vi "Live video with note capture.vi"() -> ()   [LabVIEW 2009]
uses:
  <vilib>/vision/Image Controls.llb/IMAQ Image.ctl
  <vilib>/userDefined/High Color/IMAQdx.ctl
  <vilib>/Analysis/3filter.llb/Filter Passband Type.ctl
  <vilib>/Analysis/3filter.llb/Butterworth Filter (DBL).vi
  <vilib>/vision/NI_Vision_Development_Module.lvlib
  <vilib>/Analysis/NI_AALBase.lvlib
  <vilib>/vision/driver/NI_Vision_Acquisition_Software.lvlib
panel:
  in  "frame rate":dbl
  out "Image Dst Out":T1
  out "Blue Line":T2={"Global Rectangle"=[243, 262, 261, 384], "Contours"=[{"ID"=enum."External", "Type"=2, "Coordinates"=[260, 383, 243, 262]}]} {"Contours"."Type" items=["No Selection", "Point", "Line", "Rectangle", "Oval", "Polygon", "Freehand Region", "Annulus", "Unused2", "Unused3", "Broken Line", "Freehand Line", "Rotated Rectangle"]}
  out "Red Line":T2={"Global Rectangle"=[168, 264, 180, 378], "Contours"=[{"ID"=enum."External", "Type"=2, "Coordinates"=[168, 377, 179, 264]}]} {"Contours"."Type" items=["No Selection", "Point", "Line", "Rectangle", "Oval", "Polygon", "Freehand Region", "Annulus", "Unused2", "Unused3", "Broken Line", "Freehand Line", "Rotated Rectangle"]}
  in  "low  2":dbl=0.12500000000000006 format="%0.4f"
  in  "high 2":dbl=60.0 format="%0.2f"
  in  "sampling 2":dbl=1.0 format="%0.2f"
  out "LED BLUE":bool
  out "Waveform BLUE":dbl[](graph)
  out "LED RED":bool
  in  "low":dbl=0.12500000000000006 format="%0.4f"
  out "Waveform RED":dbl[](graph)
  in  "high":dbl=60.0 format="%0.2f"
  in  "sampling":dbl=1.0 format="%0.2f"
  out "Image":T1(plugin-control)
  in  "stop":bool
  # "RED"
  # "BLUE"
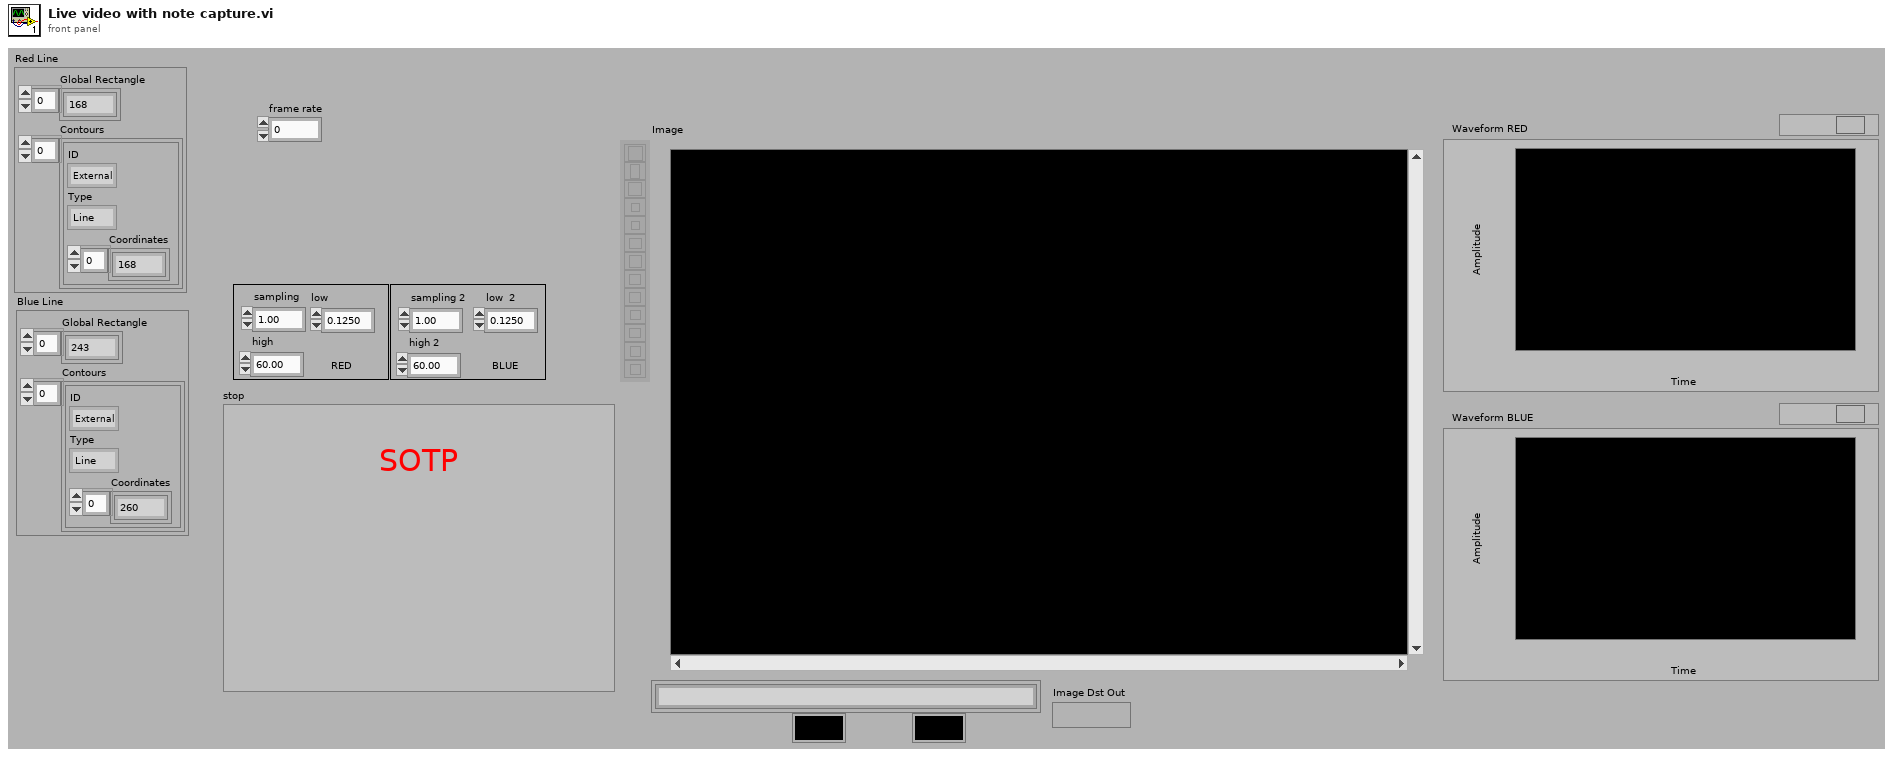
[diagram p1: front panel]
types:
  T1 = typedef "IMAQ Image.ctl" = refnum<image>
  T2 = cluster{"Global Rectangle":i32[], "Contours":cluster{"ID":enum32{"External", "Internal"}, "Type":u32, "Coordinates":i32[]}[]}
  T3 = typedef "IMAQdx.ctl" = refnum<k21>
  T4 = typedef "NI_AALBase.lvlib/Filter Passband Type.ctl" = enum32{"Lowpass", "Highpass", "Bandpass", "Bandstop"}
  T5 = cluster{"Left":i32, "Top":i32, "Right":i32, "Bottom":i32}
  T6 = typedef "Image Type" = u32
  T7 = cluster{"ID":enum32{"External", "Internal"}, "Type":u32, "Coordinates":i32[]}[]
  T8 = cluster{"ID":enum32{"External", "Internal"}, "Type":u32, "Coordinates":i32[]}
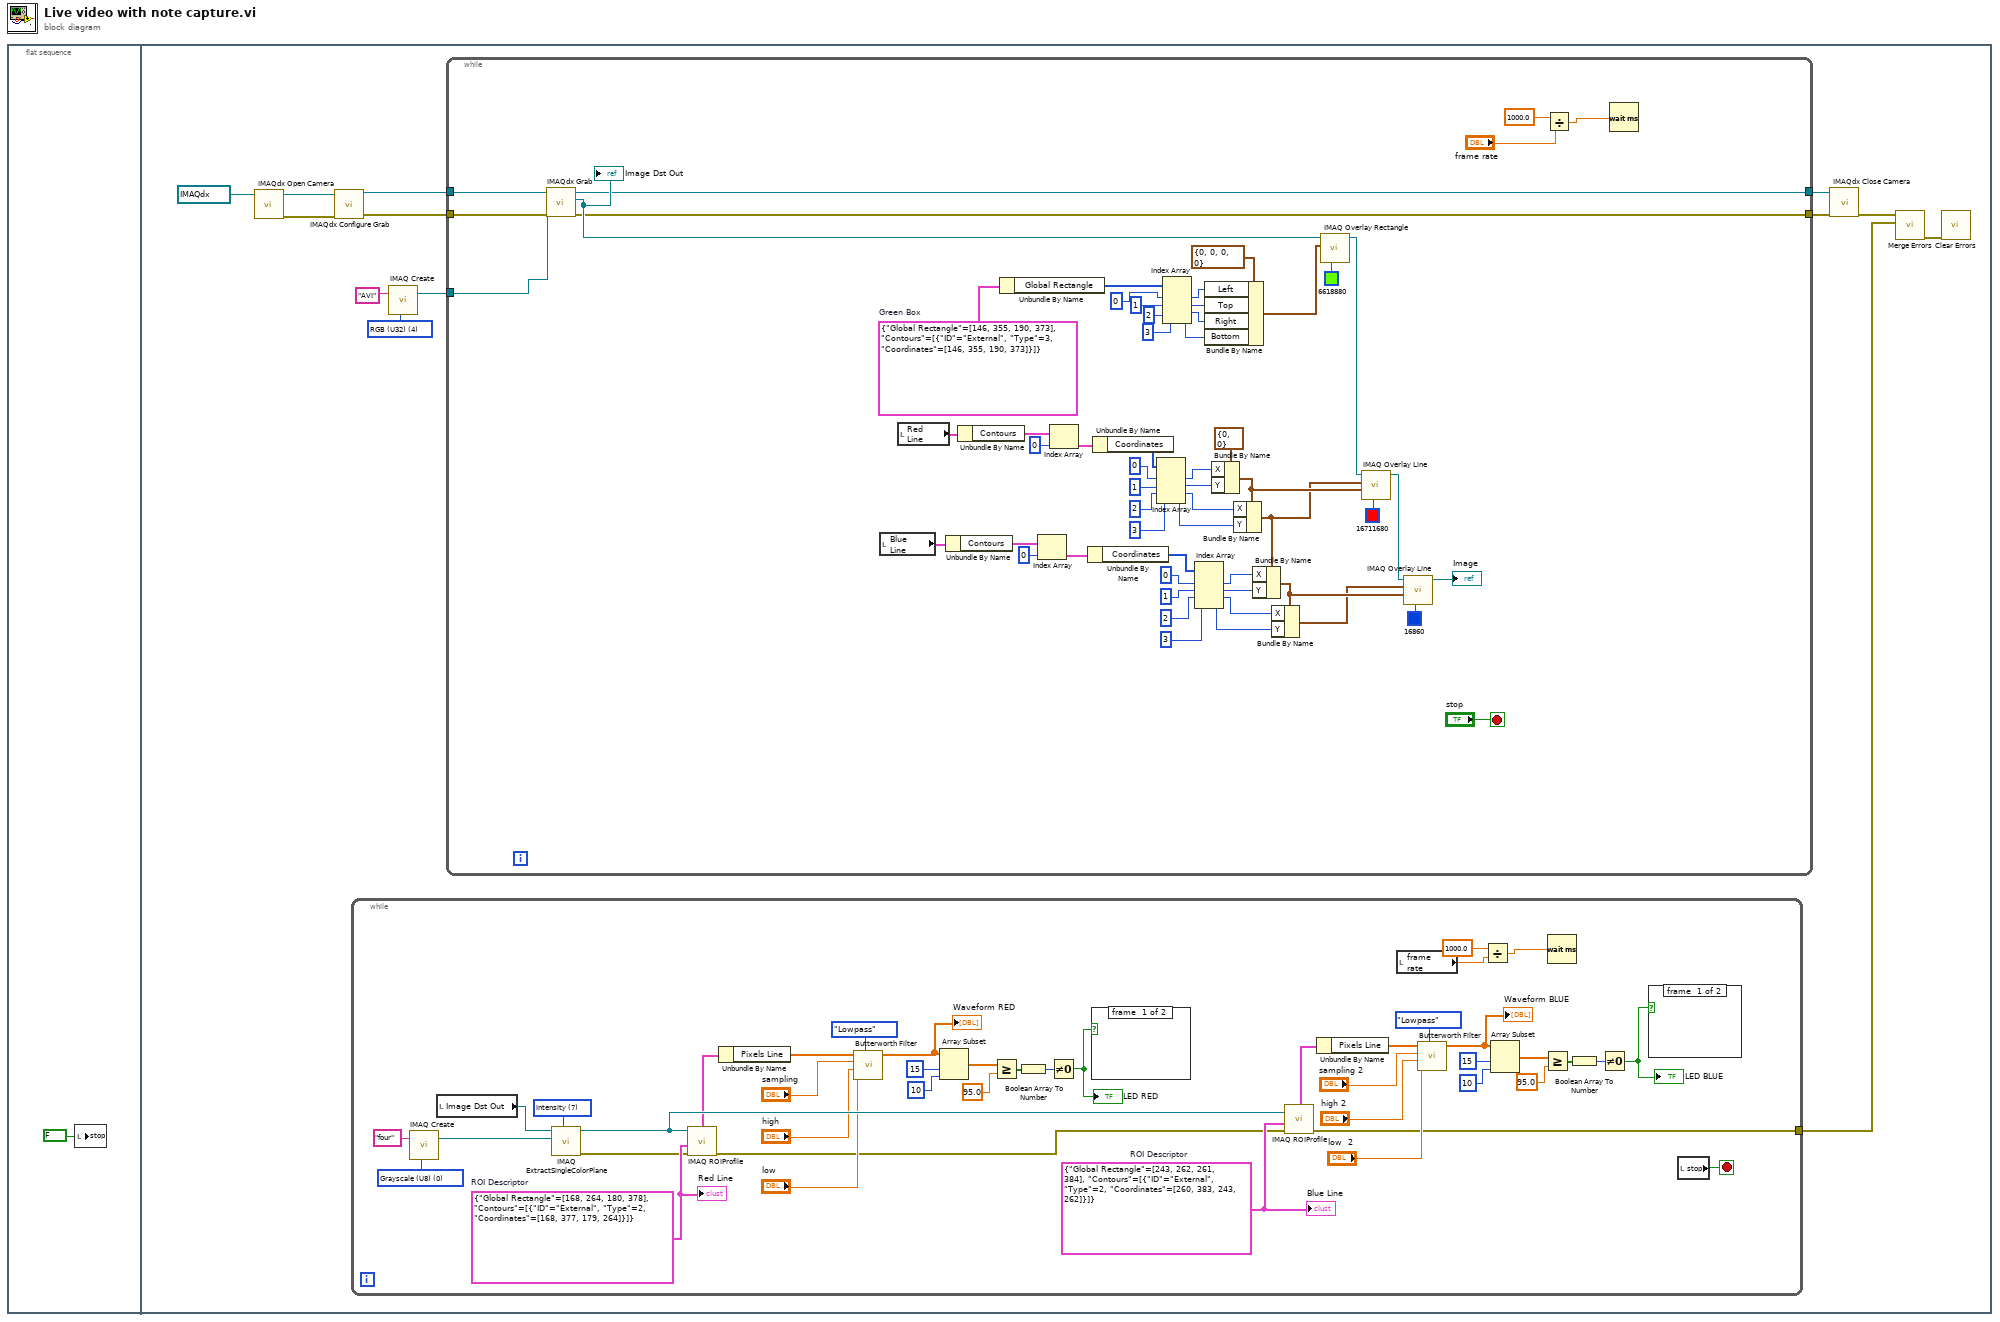
[diagram p0: block diagram]
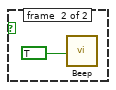
[diagram p2: hidden frame]
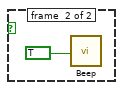
[diagram p3: hidden frame]
diagram:
  n1 = flat-sequence {
    frame #0 {
      n2 = local write "stop"(FALSE ("stop")) -> ()
    }
    frame #1 {
      w4 = T6 4 items=["Grayscale (U8)", "Grayscale (I16)", "Grayscale (SGL)", "Complex (CSG)", "RGB (U32)", "HSL (U32)", "RGB (U64)", "Grayscale (U16)"] ("Image Type")
      n3 = call <vilib>:"IMAQdx Open Camera.vi"("Session In"=T3 "cam1") -> ("error out"=w10:errorcluster, "Session Out"=w11:T3)  [unwired: 9 in]
      n4 = call <vilib>:"IMAQdx Configure Grab.vi"("error in"=w10, "Session In"=w11) -> ("error out"=w8:errorcluster, "Session Out"=w9:T3)  [unwired: 8 in]
      n5 = while {
        tunnel: [w21] -> w14
        stop <- w55 stop-if-true
        w20 = T6 0 items=["Grayscale (U8)", "Grayscale (I16)", "Grayscale (SGL)", "Complex (CSG)", "RGB (U32)", "HSL (U32)", "RGB (U64)", "Grayscale (U16)"] ("Image Type")
        w53 = T2 {"Global Rectangle"=[243, 262, 261, 384], "Contours"=[{"ID"=enum."External", "Type"=2, "Coordinates"=[260, 383, 243, 262]}]}  # ROI Descriptor
        w54 = T2 {"Global Rectangle"=[168, 264, 180, 378], "Contours"=[{"ID"=enum."External", "Type"=2, "Coordinates"=[168, 377, 179, 264]}]}  # ROI Descriptor
        w57 = 7 items=["Red", "Green", "Blue", "Hue", "Saturation", "Luminance", "Value", "Intensity"] ("Color Plane")
        n6 = call "IMAQ Create"("Image Name"="four", "Image Type"=w20) -> ("New Image"=w18:T1)  [unwired: 3 in, 1 out]
        n7 = local read "Image Dst Out"() -> (w23:T1)
        n8 = call "IMAQ ExtractSingleColorPlane"("Color Plane"=w57, "Image Dst"=w18, "Image Src"=w23) -> ("error out"=w22:errorcluster, "Image Dst Out"=w56:T1)  [unwired: 1 in, 6 out]
        n9 = call "IMAQ ROIProfile"("error in (no error)"=w22, "ROI Descriptor"=w54, "Image"=w56) -> ("error out"=w24:errorcluster, "ROI Graph"=w51:cluster{"x0":sgl, "dx":sgl, "Pixels Line":sgl[]})  [unwired: 4 out]
        n10 = Unbundle By Name(w51) -> ("Pixels Line"=w50:sgl[])
        n11 = call-poly <vilib>:"Butterworth Filter.vi"("filter type"=Filter_Passband_Type."Lowpass", "low cutoff freq: fl"="low", "high cutoff freq: fh"="high", "sampling freq: fs"="sampling", "X"=w50) -> ("Filtered X"=w46:dbl[])  [unwired: 3 in, 1 out]
        "Waveform RED" <- w46
        n12 = Array Subset(array=w46, index=15, length=10) -> (w43:dbl[])
        n13 = Greater Or Equal?(x=w43, y=95.0) -> (x >= y?=w41:bool[])
        n14 = Boolean Array To Number(Boolean array=w41) -> (number=w40:u32)
        n15 = Not Equal To 0?(x=w40) -> (x != 0?=w39:bool)
        "LED RED" <- w39
        n16 = case shown="True" w39 {
          frame #0 {
          }
          frame #1 {
            n17 = call <vilib>:"Beep.vi"("use system alert? (T)"=TRUE) -> ()  [unwired: 11 in]
          }
        }
        n18 = call "IMAQ ROIProfile"("error in (no error)"=w24, "ROI Descriptor"=w53, "Image"=w56) -> ("error out"=w21:errorcluster, "ROI Graph"=w27:cluster{"x0":sgl, "dx":sgl, "Pixels Line":sgl[]})  [unwired: 4 out]
        n19 = Unbundle By Name(w27) -> ("Pixels Line"=w30:sgl[])
        n20 = local read "frame rate"() -> (w15:dbl)
        n21 = call-poly <vilib>:"Butterworth Filter.vi"("filter type"=Filter_Passband_Type."Lowpass", "low cutoff freq: fl"="low  2", "high cutoff freq: fh"="high 2", "sampling freq: fs"="sampling 2", "X"=w30) -> ("Filtered X"=w26:dbl[])  [unwired: 3 in, 1 out]
        "Waveform BLUE" <- w26
        n22 = Divide(x=1000.0, y=w15) -> (x/y=w16:dbl)
        n23 = Array Subset(array=w26, index=15, length=10) -> (w36:dbl[])
        n24 = Greater Or Equal?(x=w36, y=95.0) -> (x >= y?=w34:bool[])
        n25 = Wait (ms)(milliseconds to wait=w16) -> ()  [unwired: 1 out]
        n26 = Boolean Array To Number(Boolean array=w34) -> (number=w33:u32)
        n27 = Not Equal To 0?(x=w33) -> (x != 0?=w32:bool)
        "LED BLUE" <- w32
        n28 = case shown="True" w32 {
          frame #0 {
          }
          frame #1 {
            n29 = call <vilib>:"Beep.vi"("use system alert? (T)"=TRUE) -> ()  [unwired: 11 in]
          }
        }
        n30 = local read "stop"() -> (w55:bool)
        "Red Line" <- w54
        "Blue Line" <- w53
      }
      n31 = call "IMAQ Create"("Image Name"="AVI", "Image Type"=w4) -> ("New Image"=w2:T1)  [unwired: 3 in, 1 out]
      n32 = while {
        tunnel: [w67] -> w5
        tunnel: [w66] -> w6
        tunnel: w9 -> [w65]
        tunnel: w8 -> [w64]
        tunnel: w2 -> [w60]
        stop <- "stop" stop-if-true
        w117 = T2 {"Global Rectangle"=[146, 355, 190, 373], "Contours"=[{"ID"=enum."External", "Type"=3, "Coordinates"=[146, 355, 190, 373]}]}  # Green Box
        n33 = call <vilib>:"IMAQdx Grab.vi"("error in"=w64, "Image In"=w60, "Session In"=w65) -> ("error out"=w66:errorcluster, "Image Out"=w68:T1, "Session Out"=w67:T3)  [unwired: 5 in, 1 out]
        "Image Dst Out" <- w68
        n34 = local read "Blue Line"() -> (w70:T2)
        n35 = local read "Red Line"() -> (w69:T2)
        n36 = Unbundle By Name(w70) -> ("Contours"=w84:T7)
        n37 = Unbundle By Name(w69) -> ("Contours"=w99:T7)
        n38 = Unbundle By Name(w117) -> ("Global Rectangle"=w113:i32[])
        n39 = Index Array(array=w84, index=0) -> (element=w83:T8)
        n40 = Index Array(array=w99, index=0) -> (element=w101:T8)
        n41 = Unbundle By Name(w83) -> ("Coordinates"=w82:i32[])
        n42 = Unbundle By Name(w101) -> ("Coordinates"=w102:i32[])
        n43 = Index Array(array=w102, index #1=0 ("index"), index #2=1 ("index"), index #3=2 ("index"), index #4=3 ("index")) -> (element #1=w94:i32, element #2=w95:i32, element #3=w96:i32, element #4=w97:i32)
        n44 = Index Array(array=w113, index #1=0 ("index"), index #2=1 ("index"), index #3=2 ("index"), index #4=3 ("index")) -> (element #1=w112:i32, element #2=w111:i32, element #3=w110:i32, element #4=w109:i32)
        n45 = Index Array(array=w82, index #1=0 ("index"), index #2=1 ("index"), index #3=2 ("index"), index #4=3 ("index")) -> (element #1=w81:i32, element #2=w87:i32, element #3=w86:i32, element #4=w85:i32)
        n46 = Bundle By Name(cluster=T5 {"Left"=0, "Top"=0, "Right"=0, "Bottom"=0} ("Rectangle"), "Left"=w112, "Top"=w111, "Right"=w110, "Bottom"=w109) -> (w115:T5)
        n47 = Bundle By Name(cluster=cluster{"X":i32, "Y":i32} {"X"=0, "Y"=0} ("End Point"), "X"=w94, "Y"=w95) -> (w103:cluster{"X":i32, "Y":i32})
        n48 = Bundle By Name(cluster=w103, "X"=w96, "Y"=w97) -> (w73:cluster{"X":i32, "Y":i32})
        n49 = Bundle By Name(cluster=w73, "X"=w81, "Y"=w87) -> (w88:cluster{"X":i32, "Y":i32})
        n50 = Bundle By Name(cluster=w88, "X"=w86, "Y"=w85) -> (w79:cluster{"X":i32, "Y":i32})
        n51 = call "IMAQ Overlay Rectangle"("Color"=u32 6618880, "Rectangle"=w115, "Image"=w68) -> ("Image Out"=w89:T1)  [unwired: 7 in, 1 out]
        n52 = call "IMAQ Overlay Line"("Color"=u32 16711680, "End Point"=w103, "Start Point"=w73, "Image"=w89) -> ("Image Out"=w78:T1)  [unwired: 6 in, 1 out]
        n53 = call "IMAQ Overlay Line"("Color"=u32 16860, "End Point"=w88, "Start Point"=w79, "Image"=w78) -> ("Image Out"=→"Image":T1)  [unwired: 6 in, 1 out]
        n54 = Divide(x=1000.0, y="frame rate") -> (x/y=w63:dbl)
        n55 = Wait (ms)(milliseconds to wait=w63) -> ()  [unwired: 1 out]
      }
      n56 = call <vilib>:"IMAQdx Close Camera.vi"("error in"=w6, "Session In"=w5) -> ("error out"=w7:errorcluster)  [unwired: 9 in]
      n57 = call <vilib>:"Merge Errors.vi"("error in 2 (no error)"=w14, "error in 1 (no error)"=w7) -> ("error out"=w13:errorcluster)  [unwired: 5 in]
      n58 = call <vilib>:"Clear Errors.vi"("error in (no error)"=w13) -> ()  [unwired: 6 in, 1 out]
    }
  }
